vi "shift_register.vi"() -> ()   [LabVIEW 2020]
panel:
  in  "stop":bool
  in  "initial num":i32
  out "result":i32
  out "iteration num":i32
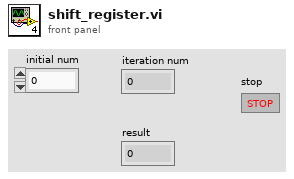
[diagram p1: front panel]
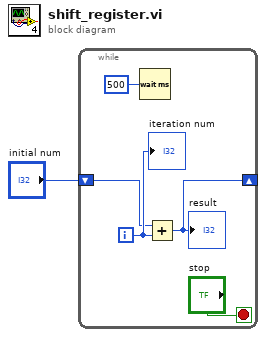
[diagram p0: block diagram]
diagram:
  n1 = while {
    shift-right: [w3] -> _
    shift-left: "initial num" -> [w4]
    i -> [w5]
    stop <- "stop" stop-if-true
    n2 = Wait (ms)(milliseconds to wait=500) -> ()  [unwired: 1 out]
    n3 = Add(x=w4, y=w5) -> (x+y=w3:i32)
    "result" <- w3
    "iteration num" <- w5
  }
